vi "My OWn PID Gyro.vi"(8 "Current Input":dbl, 10 "Wanted End":dbl, 11 "Negate Stuff":bool) -> (2 "Output":dbl, 3 "Done":bool)   [LabVIEW 2017]
uses:
  <vilib>/Rock Robotics/Network Tables/NT Write Number.vi
panel:
  # "determines what way to turn"
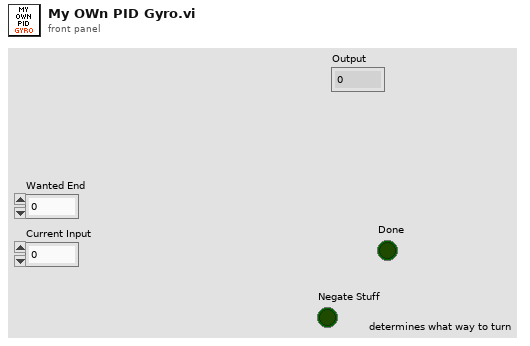
[diagram p1: front panel]
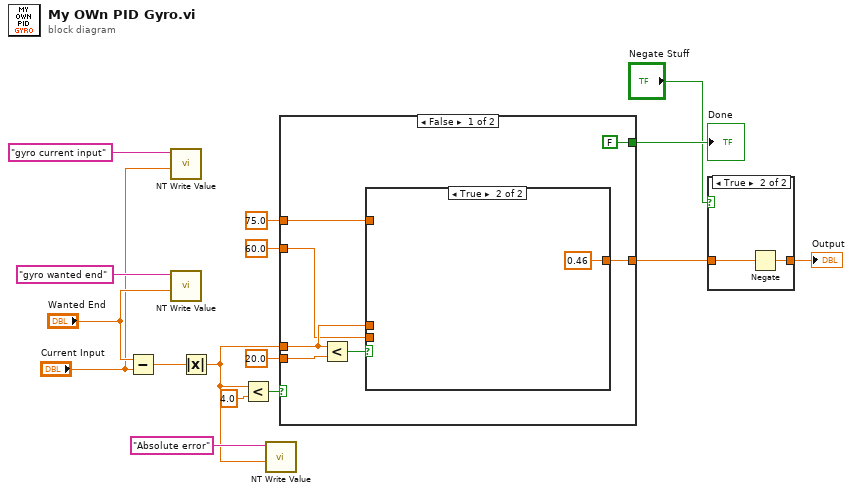
[diagram p0: block diagram]
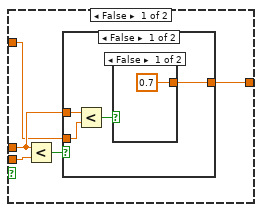
[diagram p3: hidden frame]
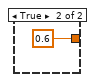
[diagram p4: hidden frame]
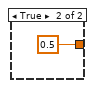
[diagram p5: hidden frame]
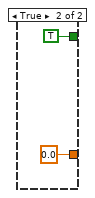
[diagram p6: hidden frame]
diagram:
  n1 = Subtract(x="Wanted End", y="Current Input") -> (x-y=w14:dbl)
  n2 = call-poly <vilib>:"NT Write Value.vi"("Numeric"="Current Input", "Name"="gyro current input") -> ()  [unwired: 9 in, 1 out]
  n3 = call-poly <vilib>:"NT Write Value.vi"("Numeric"="Wanted End", "Name"="gyro wanted end") -> ()  [unwired: 9 in, 1 out]
  n4 = Absolute Value(x=w14) -> (abs(x)=w4:dbl)
  n5 = Less?(x=w4, y=4.0) -> (x < y?=w16:bool)
  n6 = call-poly <vilib>:"NT Write Value.vi"("Numeric"=w4, "Name"="Absolute error") -> ()  [unwired: 9 in, 1 out]
  n7 = case shown="False" w16 {
    tunnel: w4 -> [w20 _]
    tunnel: [w21 0.0] -> w15
    tunnel: 20.0 -> [w23 _]
    tunnel: 60.0 -> [w19 _]
    tunnel: [FALSE TRUE] -> w10
    tunnel: 75.0 -> [w17 _]
    frame False {
      n8 = Less?(x=w20, y=w23) -> (x < y?=w22:bool)
      n9 = case shown="True" w22 {
        tunnel: [w27 0.46] -> w21
        tunnel: w20 -> [w25 _]
        tunnel: w19 -> [w28 _]
        tunnel: w17 -> [w24 _]
        frame False {
          n10 = Less?(x=w25, y=w28) -> (x < y?=w26:bool)
          n11 = case shown="False" w26 {
            tunnel: [w32 0.5] -> w27
            tunnel: w25 -> [w30 _]
            tunnel: w24 -> [w29 _]
            frame False {
              n12 = Less?(x=w30, y=w29) -> (x < y?=w31:bool)
              n13 = case shown="False" w31 {
                tunnel: [0.7 0.6] -> w32
                frame False {
                }
                frame True {
                }
              }
            }
            frame True {
            }
          }
        }
        frame True {
        }
      }
    }
    frame True {
    }
  }
  "Done" <- w10
  n14 = case shown="True" "Negate Stuff" {
    tunnel: w15 -> [w39 w41]
    tunnel: [w39 w40] -> w13
    frame False {
    }
    frame True {
      n15 = Negate(x=w41) -> (-x=w40:dbl)
    }
  }
  "Output" <- w13
